vi "Untitled 2.vi"() -> ()   [LabVIEW 2024]
panel:
  in  "Stop":bool
  out "Odd Number Indicator":bool
  out "Numeric":dbl
  in  "Start":bool
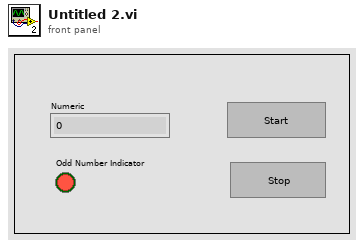
[diagram p1: front panel]
types:
  T1 = enum16{"Init", "Wait", "Start", "Odd No Chk", "Transmit", "End"}
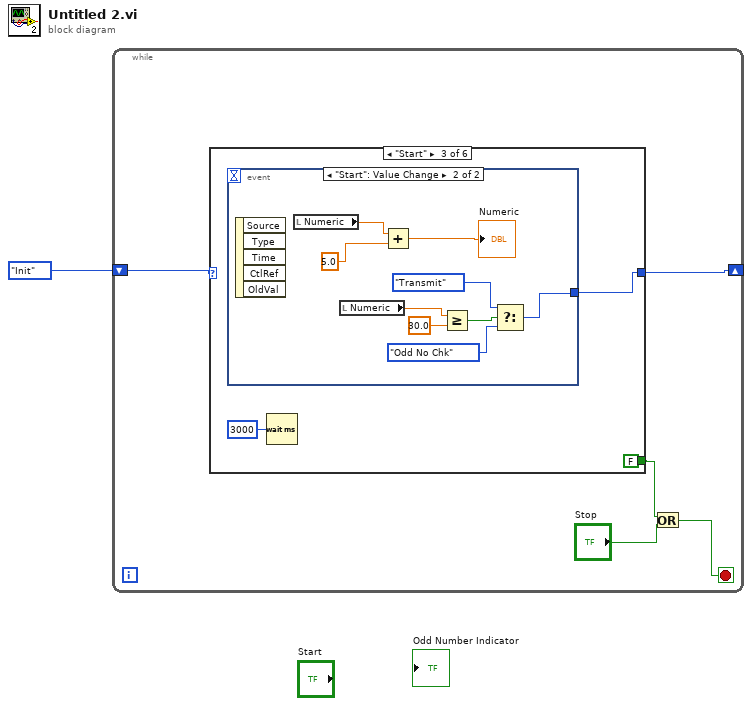
[diagram p0: block diagram]
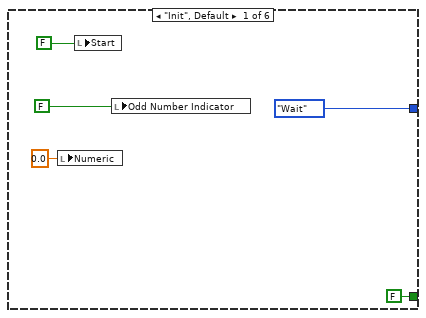
[diagram p2: hidden frame]
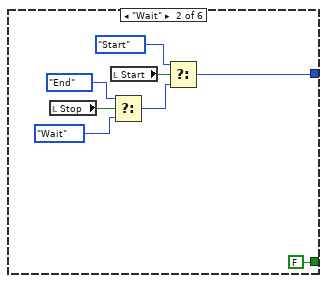
[diagram p3: hidden frame]
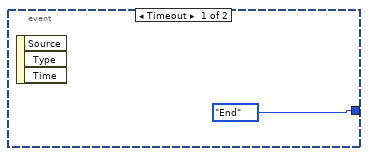
[diagram p4: hidden frame]
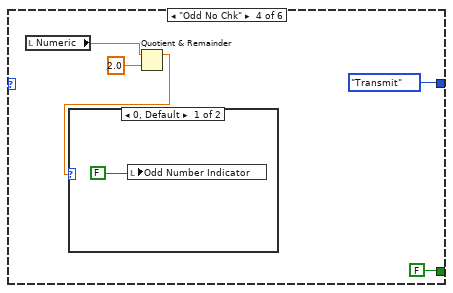
[diagram p5: hidden frame]
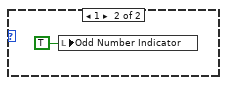
[diagram p6: hidden frame]
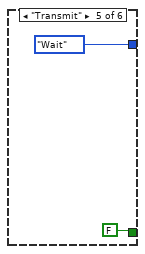
[diagram p7: hidden frame]
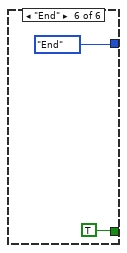
[diagram p8: hidden frame]
diagram:
  n1 = while {
    shift-right: [w5] -> _
    shift-left: T1."Init" -> [w6]
    stop <- w2 stop-if-true
    n2 = case shown="\"Start\"" w6 {
      tunnel: [_ w18 w20 T1."Transmit" T1."Wait" T1."End"] -> _
      tunnel: [T1."Wait" _ _ _ _ _] -> w5
      tunnel: [FALSE FALSE FALSE FALSE FALSE TRUE] -> w4
      frame "Init", Default {
        n3 = local write "Numeric"(0.0 ("Numeric")) -> ()
        n4 = local write "Start"(FALSE ("Stop")) -> ()
        n5 = local write "Odd Number Indicator"(FALSE ("Odd Number Indicator")) -> ()
      }
      frame "Wait" {
        n6 = local read "Stop"() -> (w16:bool)
        n7 = local read "Start"() -> (w17:bool)
        n8 = Select(t=T1."End", s=w16, f=T1."Wait") -> (s? t:f=w19:T1)
        n9 = Select(t=T1."Start", s=w17, f=w19) -> (s? t:f=w18:T1)
      }
      frame "Start" {
        n10 = event shown="[1] \"Start\": Value Change" {
          selector: _ -> [_ _]
          dyn-events: _ -> [_ _]
          timeout: _ -> [_ _]
          tunnel: [T1."End" w24] -> w20
          event Timeout {
            n11 = event-data() -> ()  [unwired: 1 in, 3 out]
          }
          event "Start": Value Change {
            n12 = event-data() -> ()  [unwired: 1 in, 5 out]
            n13 = local read "Numeric"() -> (w29:dbl)
            n14 = local read "Numeric"() -> (w31:dbl)
            n15 = Add(x=w29, y=5.0) -> (x+y=→"Numeric":dbl)
            n16 = Greater Or Equal?(x=w31, y=30.0) -> (x >= y?=w32:bool)
            n17 = Select(t=T1."Transmit", s=w32, f=T1."Odd No Chk") -> (s? t:f=w24:T1)
          }
        }
        n18 = Wait (ms)(milliseconds to wait=u32 3000) -> ()  [unwired: 1 out]
      }
      frame "Odd No Chk" {
        n19 = local read "Numeric"() -> (w36:dbl)
        n20 = Quotient & Remainder(x=w36, y=2.0) -> (x-y*floor(x/y)=w34:dbl)  [unwired: 1 out]
        n21 = case shown="0, Default" w34 {
          frame 0, Default {
            n22 = local write "Odd Number Indicator"(FALSE) -> ()
          }
          frame 1 {
            n23 = local write "Odd Number Indicator"(TRUE ("Odd Number Indicator")) -> ()
          }
        }
      }
      frame "Transmit" {
      }
      frame "End" {
      }
    }
    n24 = Or(x=w4, y="Stop") -> (x .or. y?=w2:bool)
  }
